vi "PhotonCamera_GetLEDMode.vi"(11 "CameraName":string) -> (3 "LEDMode":T1)   [LabVIEW 2019, in "PhotonVisionLib.lvlib"]
doc: "Returns the current LED mode.\n\nInputs:\n - CameraName -- The nickname of the camera (found in the PhotonVision UI).\n \nOutputs:\n - LedMode -- The current LED mode."
uses:
  PhotonVisionLib.lvlib
  TypeDef/VisionLEDModeType.ctl
  <vilib>/Rock Robotics/Network Tables/NT Read Number.vi
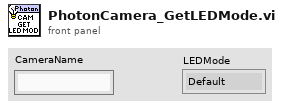
[diagram p1: front panel]
types:
  T1 = typedef "PhotonVisionLib.lvlib/VisionLEDModeType.ctl" = enum16{"Default", "Off", "On", "Blink"}
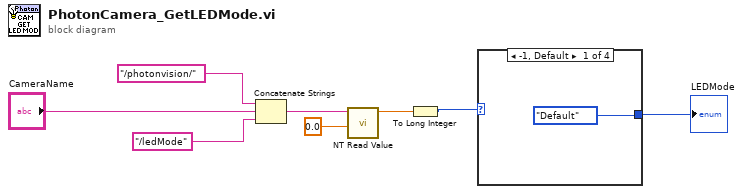
[diagram p0: block diagram]
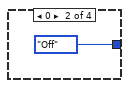
[diagram p2: hidden frame]
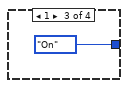
[diagram p3: hidden frame]
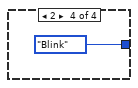
[diagram p4: hidden frame]
diagram:
  n1 = Concatenate Strings("/photonvision/", "CameraName", "/ledMode") -> (w5:string)
  n2 = call-poly <vilib>:"NT Read Value.vi"("Default Value"=0.0, "Name"=w5) -> ("Numeric"=w3:dbl)  [unwired: 8 in, 1 out]
  n3 = To Long Integer(number=w3) -> (32bit integer=w2:i32)
  n4 = case shown="-1, Default" w2 {
    tunnel: [VisionLEDModeType."Default" ("LEDMode") VisionLEDModeType."Off" ("LEDMode") VisionLEDModeType."On" ("LEDMode") VisionLEDModeType."Blink" ("LEDMode")] -> w1
    frame -1, Default {
    }
    frame 0 {
    }
    frame 1 {
    }
    frame 2 {
    }
  }
  "LEDMode" <- w1
